vi "Destroy User Events.vi"(11 "UI Template in":refnum<class "Save txt.lvclass">) -> (3 "UI Template out":refnum<class "Save txt.lvclass">)   [LabVIEW 2019, in "Save txt.lvlib" / "Save txt.lvclass"]
uses:
  Save txt.lvclass
  Save txt.lvclass/Save txt.ctl
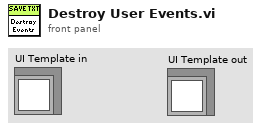
[diagram p1: front panel]
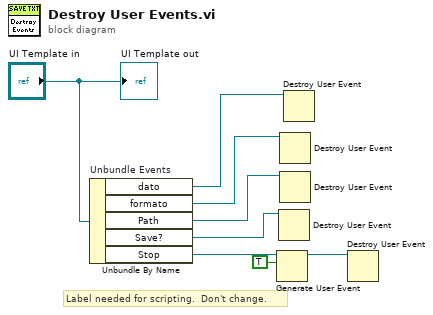
[diagram p0: block diagram]
diagram:
  # "Label needed for scripting.  Don't change."
  n1 = Unbundle By Name "Unbundle Events"("UI Template in") -> ("dato"=w1:refnum<user-event>, "formato"=w4:refnum<user-event>, "Path"=w3:refnum<user-event>, "Save?"=w2:refnum<user-event>, "Stop"=w6:refnum<user-event>)
  n2 = Generate User Event(user event=w6, event data cluster=TRUE ("event data")) -> (user event out=w7:refnum<user-event>)  [unwired: 2 in, 1 out]
  n3 = Destroy User Event(user event=w2) -> ()  [unwired: 1 in, 1 out]
  n4 = Destroy User Event(user event=w4) -> ()  [unwired: 1 in, 1 out]
  n5 = Destroy User Event(user event=w3) -> ()  [unwired: 1 in, 1 out]
  n6 = Destroy User Event(user event=w1) -> ()  [unwired: 1 in, 1 out]
  n7 = Destroy User Event(user event=w7) -> ()  [unwired: 1 in, 1 out]
  "UI Template out" <- "UI Template in"
